vi "Calculate_orientation_student.vi"(9 "IMU_in":dbl[](array[numeric]), 11 "Reset":bool) -> (3 "Orientation (pitch, roll, yaw)":dbl[](array[numeric]))   [LabVIEW 2014]
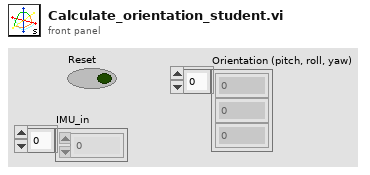
[diagram p1: front panel]
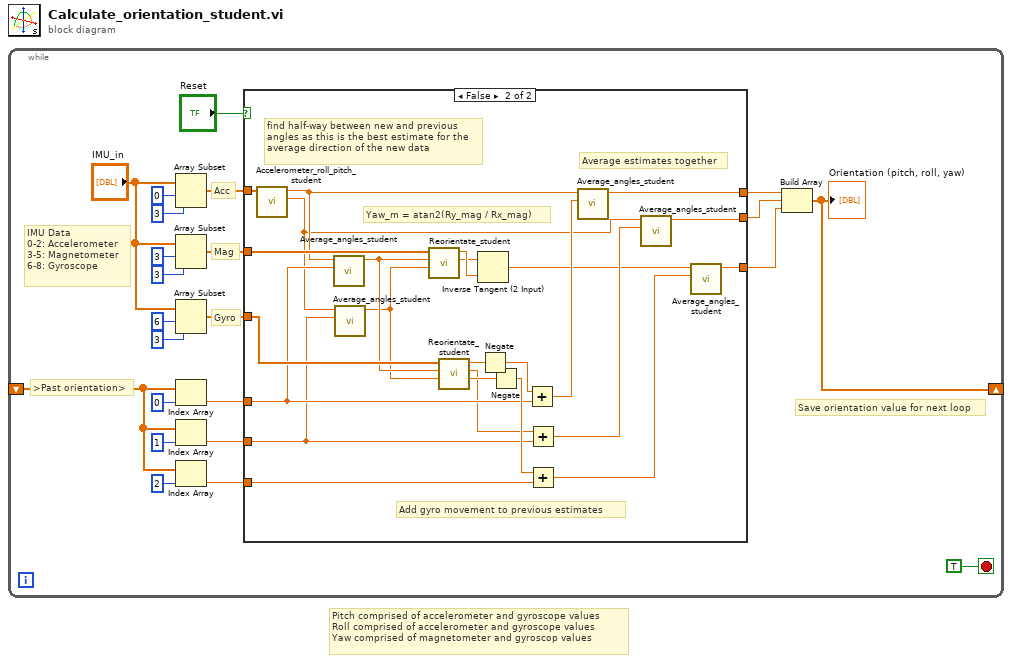
[diagram p0: block diagram]
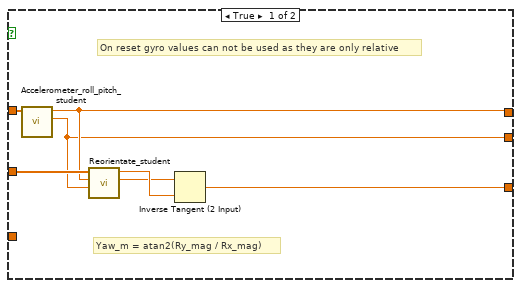
[diagram p2: hidden frame]
diagram:
  # "Pitch comprised of accelerometer and gyroscope values\nRoll comprised of accelerometer and gyroscope values\nYaw comprised of magnetometer and gyroscop values"
  n1 = while {
    shift-right: [w2] -> _
    shift-left: _ -> [w1]
    stop <- TRUE stop-if-true
    # "Save orientation value for next loop"
    # "Gyro"
    # "Mag"
    # "Acc"
    # ">Past orientation>"
    # "IMU Data\n0-2: Accelerometer\n3-5: Magnetometer\n6-8: Gyroscope"
    n2 = Array Subset(array="IMU_in", index=0, length=3) -> (w14:dbl[])
    n3 = Array Subset(array="IMU_in", index=3, length=3) -> (w19:dbl[])
    n4 = Array Subset(array="IMU_in", index=6, length=3) -> (w18:dbl[])
    n5 = Index Array(array=w1, index=0) -> (element=w9:dbl)
    n6 = Index Array(array=w1, index=1) -> (element=w8:dbl)
    n7 = Index Array(array=w1, index=2) -> (element=w7:dbl)
    n8 = case shown="False" "Reset" {
      tunnel: w19 -> [w28 w52]
      tunnel: w18 -> [_ w48]
      tunnel: w14 -> [w27 w51]
      tunnel: [w26 w44] -> w6
      tunnel: [w25 w41] -> w5
      tunnel: [w24 w40] -> w4
      tunnel: w9 -> [_ w36]
      tunnel: w8 -> [_ w33]
      tunnel: w7 -> [_ w45]
      frame True {
        # "On reset gyro values can not be used as they are only relative"
        # "Yaw_m = atan2(Ry_mag / Rx_mag)"
        n9 = call "Accelerometer_roll_pitch_student.vi"("Accelerometer Data (x, y, z)"=w27) -> ("Roll_a"=w25:dbl, "Pitch_a"=w26:dbl)  [unwired: 9 in]
        n10 = call "Reorientate_student.vi"("Roll"=w25, "Pitch"=w26, "Vector (x, y, z)"=w28) -> ("Ry"=w29:dbl, "Rx"=w30:dbl)  [unwired: 6 in, 1 out]
        n11 = Inverse Tangent (2 Input)(1:w30, 2:w29) -> (0:w24:dbl)
      }
      frame False {
        # "Yaw_m = atan2(Ry_mag / Rx_mag)"
        # "Add gyro movement to previous estimates"
        # "Average estimates together"
        # "find half-way between new and previous\nangles as this is the best estimate for the\naverage direction of the new data"
        n12 = call "Accelerometer_roll_pitch_student.vi"("Accelerometer Data (x, y, z)"=w51) -> ("Roll_a"=w34:dbl, "Pitch_a"=w37:dbl)  [unwired: 9 in]
        n13 = call "Average_angles_student.vi"("Angle_2"=w36, "Angle_1"=w37) -> ("Angle_average"=w35:dbl)  [unwired: 9 in]
        n14 = call "Average_angles_student.vi"("Angle_2"=w33, "Angle_1"=w34) -> ("Angle_average"=w32:dbl)  [unwired: 9 in]
        n15 = call "Reorientate_student.vi"("Roll"=w32, "Pitch"=w35, "Vector (x, y, z)"=w52) -> ("Ry"=w53:dbl, "Rx"=w54:dbl)  [unwired: 6 in, 1 out]
        n16 = call "Reorientate_student.vi"("Roll"=w32, "Pitch"=w35, "Vector (x, y, z)"=w48) -> ("Rz"=w49:dbl, "Ry"=w31:dbl, "Rx"=w50:dbl)  [unwired: 6 in]
        n17 = Inverse Tangent (2 Input)(1:w54, 2:w53) -> (0:w39:dbl)
        n18 = Negate(x=w50) -> (-x=w47:dbl)
        n19 = Negate(x=w49) -> (-x=w46:dbl)
        n20 = Add(x=w47, y=w36) -> (x+y=w43:dbl)
        n21 = Add(x=w31, y=w33) -> (x+y=w42:dbl)
        n22 = Add(x=w46, y=w45) -> (x+y=w38:dbl)
        n23 = call "Average_angles_student.vi"("Angle_2"=w43, "Angle_1"=w37) -> ("Angle_average"=w44:dbl)  [unwired: 9 in]
        n24 = call "Average_angles_student.vi"("Angle_2"=w42, "Angle_1"=w34) -> ("Angle_average"=w41:dbl)  [unwired: 9 in]
        n25 = call "Average_angles_student.vi"("Angle_2"=w38, "Angle_1"=w39) -> ("Angle_average"=w40:dbl)  [unwired: 9 in]
      }
    }
    n26 = Build Array(w6, w5, w4) -> (w2:dbl[])
    "Orientation (pitch, roll, yaw)" <- w2
  }
